vi "Parse test.vi"() -> ()   [LabVIEW 2025]
uses:
  <vilib>/Utility/error.llb/Trim Whitespace One-Sided.vi
panel:
  in  "Energy":string="220.000000,221.000000,223.000000; 50.000000,50.100000,50.200000; 10.100000,10.200000,10.300000; 1.100000,1.200000,1.300000; 0\n\n"
  in  "Power":string="220.000000,221.000000,223.000000; 50.000000,50.100000,50.200000; 10.100000,10.200000,10.300000; 1.100000,1.200000,1.300000; 0\n\n"
  out "PSU Values 3PH":T1
  out "PSU Values":T2
  in  "Basic  quantities":string="220.000000,221.000000,223.000000; 50.000000,50.100000,50.200000; 10.100000,10.200000,10.300000; 1.100000,1.200000,1.300000; 0\n\n"
  # "In 3phase system values are \naverage of all three phases"
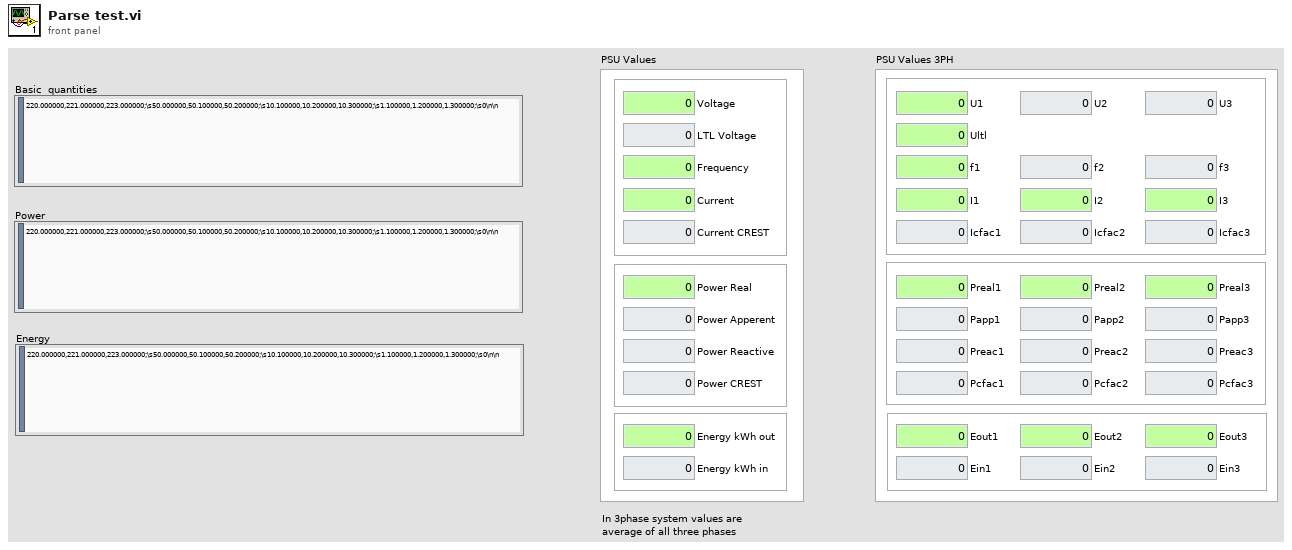
[diagram p1: front panel]
types:
  T1 = cluster{"U1":dbl, "U2":dbl, "U3":dbl, "Ultl":dbl, "f1":dbl, "f2":dbl, "f3":dbl, "I1":dbl, "I2":dbl, "I3":dbl, "Icfac1":dbl, "Icfac2":dbl, "Icfac3":dbl, "Preal1":dbl, "Preal2":dbl, "Preal3":dbl, "Papp1":dbl, "Papp2":dbl, "Papp3":dbl, "Preac1":dbl, "Preac2":dbl, "Preac3":dbl, "Pcfac1":dbl, "Pcfac2":dbl, "Pcfac3":dbl, "Eout1":dbl, "Eout2":dbl, "Eout3":dbl, "Ein1":dbl, "Ein2":dbl, "Ein3":dbl}
  T2 = cluster{"Voltage":dbl, "LTL Voltage":dbl, "Current":dbl, "Current CREST":dbl, "Power Real":dbl, "Power Apperent":dbl, "Power Reactive":dbl, "Power CREST":dbl, "Energy kWh out":dbl, "Energy kWh in":dbl, "Frequency":dbl}
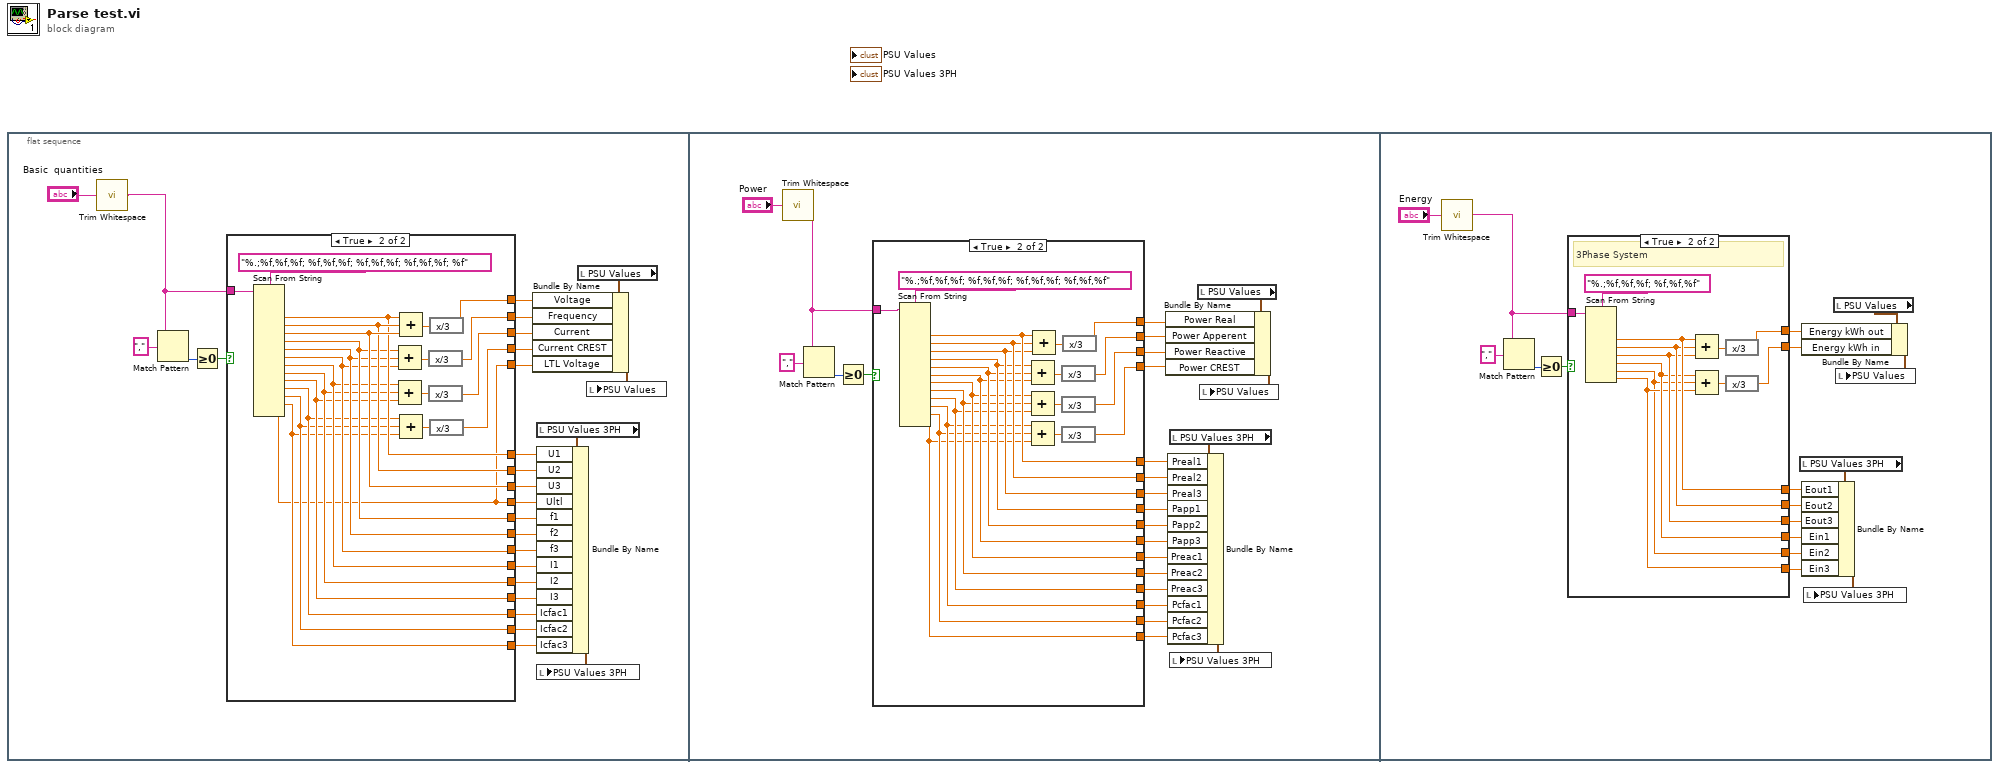
[diagram p0: block diagram]
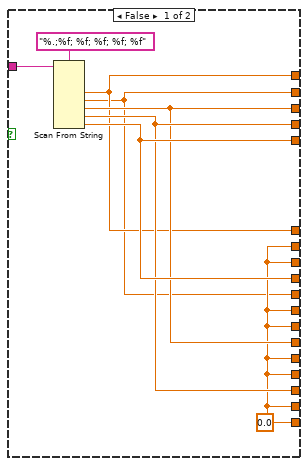
[diagram p2: hidden frame]
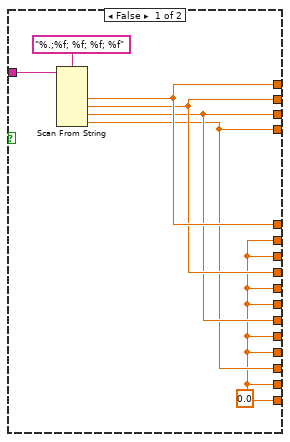
[diagram p3: hidden frame]
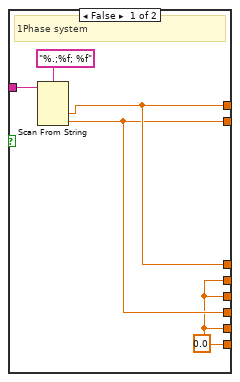
[diagram p4: hidden frame]
diagram:
  n1 = flat-sequence {
    frame #0 {
      n2 = call <vilib>:"Trim Whitespace.vi"("string"="Basic  quantities") -> ("trimmed string"=w1:string)  [unwired: 1 in]
      n3 = Match Pattern(string=w1, regular expression=",") -> (offset past match=w18:i32)  [unwired: 1 in, 3 out]
      n4 = Greater Or Equal To 0?(x=w18) -> (x >= 0?=w17:bool)
      n5 = case shown="True" w17 {
        tunnel: [w29 w48] -> w26
        tunnel: [w28 w47] -> w25
        tunnel: [w31 w42] -> w24
        tunnel: [w32 w40] -> w23
        tunnel: [w33 w36] -> w21
        tunnel: w1 -> [w34 w58]
        tunnel: [w29 w54] -> w14
        tunnel: [w30 w55] -> w13
        tunnel: [w30 w56] -> w12
        tunnel: [w33 w36] -> w11
        tunnel: [w28 w51] -> w10
        tunnel: [w30 w50] -> w9
        tunnel: [w30 w49] -> w8
        tunnel: [w31 w45] -> w7
        tunnel: [w30 w44] -> w6
        tunnel: [w30 w43] -> w5
        tunnel: [w32 w39] -> w4
        tunnel: [w30 w38] -> w3
        tunnel: [w30 w37] -> w2
        frame False {
          w30 = 0.0
          n6 = Scan From String(format string="%.;%f; %f; %f; %f; %f", input string=w34) -> (output 1=w29:dbl, output 2=w28:dbl, output 3=w31:dbl, output 4=w32:dbl, output 5=w33:dbl)  [unwired: 7 in, 3 out]
        }
        frame True {
          n7 = Scan From String(format string="%.;%f,%f,%f; %f,%f,%f; %f,%f,%f; %f,%f,%f; %f", input string=w58) -> (output 1=w54:dbl, output 2=w55:dbl, output 3=w56:dbl, output 4=w51:dbl, output 5=w50:dbl, output 6=w49:dbl, output 7=w45:dbl, output 8=w44:dbl, output 9=w43:dbl, output 10=w39:dbl, output 11=w38:dbl, output 12=w37:dbl, output 13=w36:dbl)  [unwired: 15 in, 3 out]
          n8 = Compound Arithmetic op=ADD(w51, w50, w49) -> (w52:dbl)
          n9 = Compound Arithmetic op=ADD(w45, w44, w43) -> (w46:dbl)
          n10 = Compound Arithmetic op=ADD(w54, w55, w56) -> (w53:dbl)
          n11 = Compound Arithmetic op=ADD(w39, w38, w37) -> (w41:dbl)
          n12 = expression code="x/3"(w52) -> (w47:dbl)
          n13 = expression code="x/3"(w46) -> (w42:dbl)
          n14 = expression code="x/3"(w53) -> (w48:dbl)
          n15 = expression code="x/3"(w41) -> (w40:dbl)
        }
      }
      n16 = local read "PSU Values 3PH"() -> (w16:T1)
      n17 = Bundle By Name(cluster=w16, "U1"=w14, "U2"=w13, "U3"=w12, "Ultl"=w11, "f1"=w10, "f2"=w9, "f3"=w8, "I1"=w7, "I2"=w6, "I3"=w5, "Icfac1"=w4, "Icfac2"=w3, "Icfac3"=w2) -> (w15:T1)
      n18 = local write "PSU Values 3PH"(w15) -> ()
      n19 = local read "PSU Values"() -> (w27:T2)
      n20 = Bundle By Name(cluster=w27, "Voltage"=w26, "Frequency"=w25, "Current"=w24, "Current CREST"=w23, "LTL Voltage"=w21) -> (w22:T2)
      n21 = local write "PSU Values"(w22) -> ()
    }
    frame #1 {
      n22 = call <vilib>:"Trim Whitespace.vi"("string"="Power") -> ("trimmed string"=w67:string)  [unwired: 1 in]
      n23 = Match Pattern(string=w67, regular expression=",") -> (offset past match=w60:i32)  [unwired: 1 in, 3 out]
      n24 = Greater Or Equal To 0?(x=w60) -> (x >= 0?=w61:bool)
      n25 = case shown="True" w61 {
        tunnel: [w88 w94] -> w63
        tunnel: [w87 w93] -> w64
        tunnel: [w86 w92] -> w65
        tunnel: [w85 w91] -> w66
        tunnel: w67 -> [w89 w112]
        tunnel: [w88 w109] -> w72
        tunnel: [w87 w105] -> w73
        tunnel: [w86 w102] -> w74
        tunnel: [w85 w97] -> w75
        tunnel: [w84 w95] -> w76
        tunnel: [w84 w96] -> w77
        tunnel: [w84 w100] -> w78
        tunnel: [w84 w101] -> w79
        tunnel: [w84 w103] -> w80
        tunnel: [w84 w104] -> w81
        tunnel: [w84 w107] -> w82
        tunnel: [w84 w108] -> w83
        frame False {
          w84 = 0.0
          n26 = Scan From String(format string="%.;%f; %f; %f; %f", input string=w89) -> (output 1=w88:dbl, output 2=w87:dbl, output 3=w86:dbl, output 4=w85:dbl)  [unwired: 6 in, 3 out]
        }
        frame True {
          n27 = Scan From String(format string="%.;%f,%f,%f; %f,%f,%f; %f,%f,%f; %f,%f,%f", input string=w112) -> (output 1=w109:dbl, output 2=w108:dbl, output 3=w107:dbl, output 4=w105:dbl, output 5=w104:dbl, output 6=w103:dbl, output 7=w102:dbl, output 8=w101:dbl, output 9=w100:dbl, output 10=w97:dbl, output 11=w96:dbl, output 12=w95:dbl)  [unwired: 14 in, 3 out]
          n28 = Compound Arithmetic op=ADD(w105, w104, w103) -> (w106:dbl)
          n29 = Compound Arithmetic op=ADD(w102, w101, w100) -> (w98:dbl)
          n30 = Compound Arithmetic op=ADD(w97, w96, w95) -> (w99:dbl)
          n31 = Compound Arithmetic op=ADD(w109, w108, w107) -> (w110:dbl)
          n32 = expression code="x/3"(w106) -> (w93:dbl)
          n33 = expression code="x/3"(w98) -> (w92:dbl)
          n34 = expression code="x/3"(w99) -> (w91:dbl)
          n35 = expression code="x/3"(w110) -> (w94:dbl)
        }
      }
      n36 = local read "PSU Values 3PH"() -> (w71:T1)
      n37 = Bundle By Name(cluster=w71, "Preal1"=w72, "Preal2"=w83, "Preal3"=w82, "Papp1"=w73, "Papp2"=w81, "Papp3"=w80, "Preac1"=w74, "Preac2"=w79, "Preac3"=w78, "Pcfac1"=w75, "Pcfac2"=w77, "Pcfac3"=w76) -> (w70:T1)
      n38 = local write "PSU Values 3PH"(w70) -> ()
      n39 = local read "PSU Values"() -> (w69:T2)
      n40 = Bundle By Name(cluster=w69, "Power Real"=w63, "Power Apperent"=w64, "Power Reactive"=w65, "Power CREST"=w66) -> (w68:T2)
      n41 = local write "PSU Values"(w68) -> ()
    }
    frame #2 {
      n42 = call <vilib>:"Trim Whitespace.vi"("string"="Energy") -> ("trimmed string"=w126:string)  [unwired: 1 in]
      n43 = Match Pattern(string=w126, regular expression=",") -> (offset past match=w127:i32)  [unwired: 1 in, 3 out]
      n44 = Greater Or Equal To 0?(x=w127) -> (x >= 0?=w125:bool)
      n45 = case shown="True" w125 {
        tunnel: w126 -> [w133 w146]
        tunnel: [w132 w136] -> w124
        tunnel: [w131 w135] -> w123
        tunnel: [w132 w142] -> w118
        tunnel: [w131 w139] -> w117
        tunnel: [w130 w138] -> w116
        tunnel: [w130 w137] -> w115
        tunnel: [w130 w140] -> w114
        tunnel: [w130 w141] -> w113
        frame False {
          w130 = 0.0
          # "1Phase system"
          n46 = Scan From String(format string="%.;%f; %f", input string=w133) -> (output 1=w132:dbl, output 2=w131:dbl)  [unwired: 4 in, 3 out]
        }
        frame True {
          # "3Phase System"
          n47 = Scan From String(format string="%.;%f,%f,%f; %f,%f,%f", input string=w146) -> (output 1=w142:dbl, output 2=w141:dbl, output 3=w140:dbl, output 4=w139:dbl, output 5=w137:dbl, output 6=w138:dbl)  [unwired: 8 in, 3 out]
          n48 = Compound Arithmetic op=ADD(w142, w141, w140) -> (w144:dbl)
          n49 = Compound Arithmetic op=ADD(w139, w137, w138) -> (w143:dbl)
          n50 = expression code="x/3"(w144) -> (w136:dbl)
          n51 = expression code="x/3"(w143) -> (w135:dbl)
        }
      }
      n52 = local read "PSU Values 3PH"() -> (w120:T1)
      n53 = Bundle By Name(cluster=w120, "Eout1"=w118, "Eout2"=w113, "Eout3"=w114, "Ein1"=w117, "Ein2"=w115, "Ein3"=w116) -> (w119:T1)
      n54 = local write "PSU Values 3PH"(w119) -> ()
      n55 = local read "PSU Values"() -> (w122:T2)
      n56 = Bundle By Name(cluster=w122, "Energy kWh out"=w124, "Energy kWh in"=w123) -> (w121:T2)
      n57 = local write "PSU Values"(w121) -> ()
    }
  }
